vi "time calc.vi"(0 "millisecond timer value":u32, 7 "system state in":T1) -> (8 "system state out":T1)   [LabVIEW 2016]
doc: "This Vi calculates the the current time and time remaining based on the state time, and outputs the new time.\n\nAlexis Lopez\nP350\nCSUSB Physics"
uses:
  typedefs/system state cluster.ctl
  typedefs/state enum.ctl
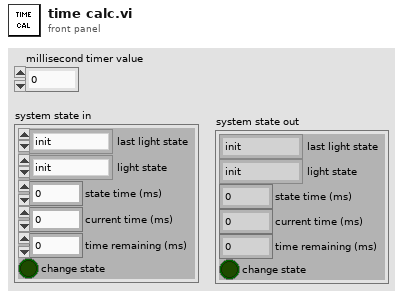
[diagram p1: front panel]
types:
  T1 = typedef "system state cluster.ctl" = cluster{"last light state":T2, "light state":T2, "state time (ms)":i32, "current time (ms)":i32, "time remaining (ms)":i32, "change state":bool}
  T2 = typedef "state enum.ctl" = enum16{"init", "idle", "left turn E", "go EW", "caution EW", "left turn W", "left turn N", "go NS", "caution NS", "left turn S", "blink on", "blink off", "all on test", "exit"}
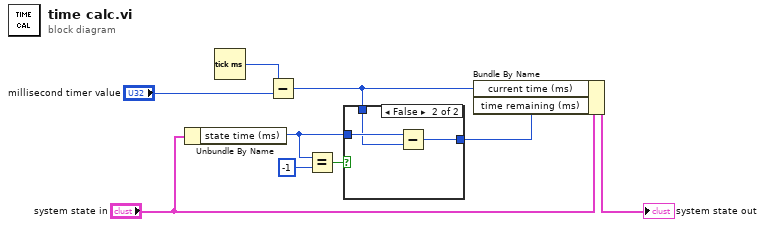
[diagram p0: block diagram]
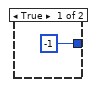
[diagram p2: hidden frame]
diagram:
  n1 = Unbundle By Name("system state in") -> ("state time (ms)"=w2:i32)
  n2 = Tick Count (ms)() -> (millisecond timer value=w9:u32)
  n3 = Subtract(x=w9, y="millisecond timer value") -> (x-y=w5:u32)
  n4 = Equal?(x=w2, y=-1) -> (x = y?=w3:bool)
  n5 = case shown="False" w3 {
    tunnel: w2 -> [_ w13]
    tunnel: w5 -> [_ w12]
    tunnel: [-1 w11] -> w4
    frame True {
    }
    frame False {
      n6 = Subtract(x=w13, y=w12) -> (x-y=w11:u32)
    }
  }
  n7 = Bundle By Name(cluster="system state in", "current time (ms)"=w5, "time remaining (ms)"=w4) -> (→"system state out":T1)
